vi "CAN Get Value.vi"   [LabVIEW 2020, in "PCANBasic.lvlib"]
doc: "Retrieves information from a PCAN Channel.\n\nParameters Description \nChannel The handle of a PCAN Channel (see TPCANHandle). \nParameter The code of the information to be retrieved. \nBuffer The buffer to return the required value. \nBufferLength The length in bytes of the given buffer. \n\nReturns:\nInputs and outputs of this Vi depend on the selected function.\nThe instances of the VI are in the Get Value path."
uses:
  <userlib>/PCAN Basic/PCANBasic.lvlib
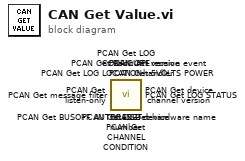
[diagram p0: block diagram]
diagram:
  n1 = call <userlib>:"PCAN Get USB device number.vi"() -> ()  [unwired: 9 in, 3 out]
  n2 = call <userlib>:"PCAN Get receive event handler .vi"() -> ()  [unwired: 9 in, 3 out]
  n3 = call <userlib>:"PCAN Get message filter.vi"() -> ()  [unwired: 9 in, 3 out]
  n4 = call <userlib>:"PCAN Get LOG STATUS.vi"() -> ()  [unwired: 9 in, 3 out]
  n5 = call <userlib>:"PCAN Get LOG LOCATION.vi"() -> ()  [unwired: 9 in, 3 out]
  n6 = call <userlib>:"PCAN Get LOG CONFIGURE.vi"() -> ()  [unwired: 9 in, 3 out]
  n7 = call <userlib>:"PCAN Get listen-only.vi"() -> ()  [unwired: 9 in, 3 out]
  n8 = call <userlib>:"PCAN Get hardware name.vi"() -> ()  [unwired: 9 in, 3 out]
  n9 = call <userlib>:"PCAN Get device channel version.vi"() -> ()  [unwired: 9 in, 3 out]
  n10 = call <userlib>:"PCAN Get CHANNEL CONDITION.vi"() -> ()  [unwired: 9 in, 3 out]
  n11 = call <userlib>:"PCAN Get BUSOFF AUTORESET.vi"() -> ()  [unwired: 9 in, 3 out]
  n12 = call <userlib>:"PCAN Get Basic API version.vi"() -> ()  [unwired: 10 in, 2 out]
  n13 = call <userlib>:"PCAN Get 5VOLTS POWER.vi"() -> ()  [unwired: 9 in, 3 out]
